vi "Date to Dir Name (old).vi"() -> (0 "Dir Name":string)   [LabVIEW 2015, in "File IO.lvclass"]
uses:
  File IO.lvclass
panel:
  out "Year":string
  out "Day":string
  out "Month":string
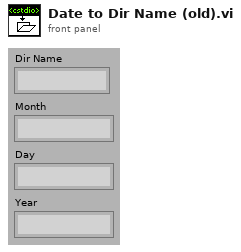
[diagram p1: front panel]
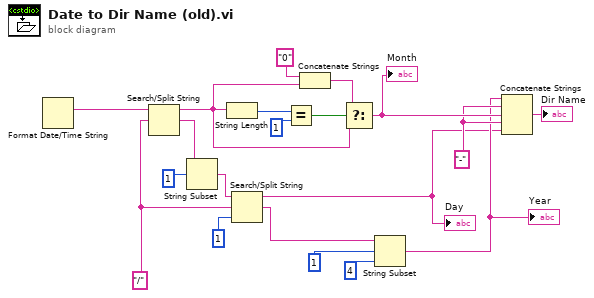
[diagram p0: block diagram]
diagram:
  w6 = "-"
  w14 = "/"
  n1 = Format Date/Time String() -> (date/time string=w20:string)  [unwired: 3 out]
  n2 = Search/Split String(string=w20, search string/char (-)=w14) -> (substring before match=w9:string, match + rest of string=w3:string)  [unwired: 2 out]
  n3 = String Subset(string=w3, offset (0)=1) -> (substring=w1:string)  [unwired: 1 out]
  n4 = String Length(string=w9) -> (length=w19:i32)
  n5 = Search/Split String(string=w1, search string/char (-)=w14, offset (0)=1) -> (substring before match=w4:string, match + rest of string=w13:string)  [unwired: 1 out]
  "Day" <- w4
  n6 = Equal?(x=w19, y=1) -> (x = y?=w16:bool)
  n7 = Concatenate Strings("0", w9) -> (w15:string)
  n8 = Select(t=w15, s=w16, f=w9) -> (s? t:f=w10:string)
  "Month" <- w10
  n9 = String Subset(string=w13, offset (0)=1, length (rest)=4) -> (substring=w5:string)
  "Year" <- w5
  n10 = Concatenate Strings(w5, w6, w10, w6, w4) -> (→"Dir Name":string)
